vi "Cluster_Example.vi"(11 "Cluster":T1) -> (3 "output cluster":T1)   [LabVIEW 2024]
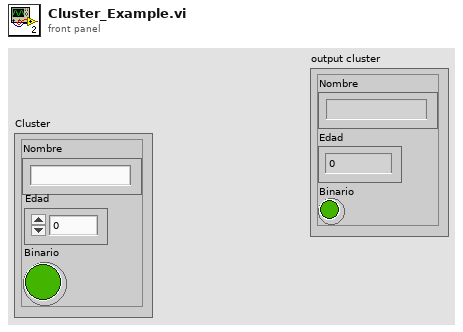
[diagram p1: front panel]
types:
  T1 = cluster{"Nombre":string, "Edad":dbl, "Binario":bool}
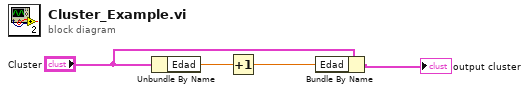
[diagram p0: block diagram]
diagram:
  n1 = Unbundle By Name("Cluster") -> ("Edad"=w4:dbl)
  n2 = Increment(x=w4) -> (x+1=w2:dbl)
  n3 = Bundle By Name(cluster="Cluster", "Edad"=w2) -> (→"output cluster":T1)
